vi "Asia Pump C Test.vi"() -> ()   [LabVIEW 2018, in "ASIA Pump.lvlib"]
uses:
  ASIA Pump.lvlib
  ASIA Pump/Pump Settings.ctl
panel:
  out "ASIA Pump Global 2":T1(array[cluster])
  out "Pump On?":enum16{"Off", "On", "Not Initialized"}(ring)
  out "pressure":dbl
  out "Connection Error 2":bool
  out "Connection Error":bool
  out "Pump Status Time":dbl
  out "Set Speed Time":dbl
  in  "Pump %":sgl
  in  "stop":bool
  out "PumpStatusCode":T2(ring)=enum."Idle"
  out "pumpRate":dbl format="%.2f"
  out "syringeSize":sgl
  in  "Run":bool
  in  "ASIA Pump C Settings in":T3
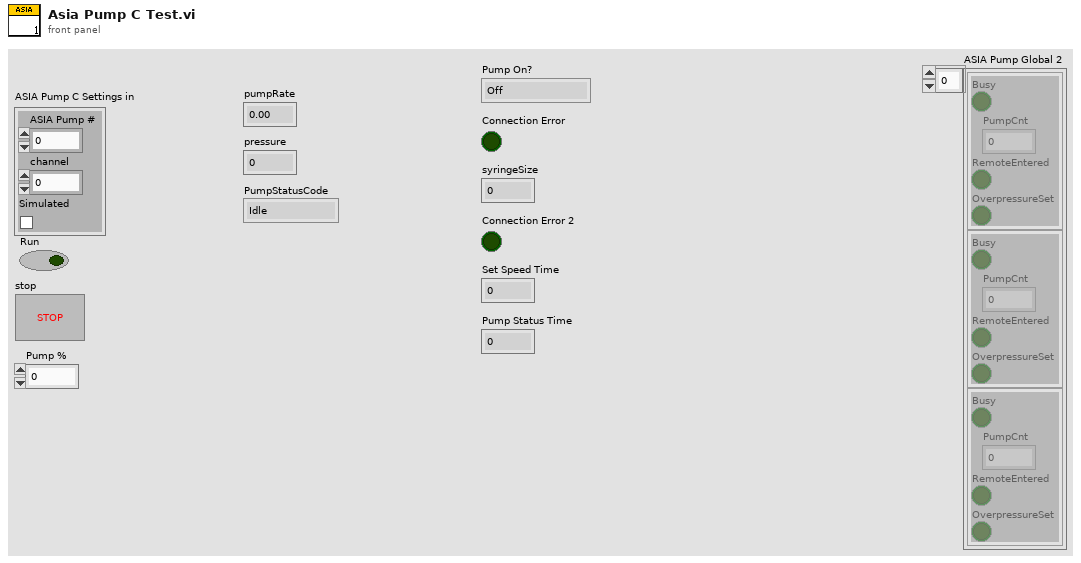
[diagram p1: front panel]
types:
  T1 = cluster{"Busy":bool, "PumpCnt":dbl, "RemoteEntered":bool, "OverpressureSet":bool}[]
  T2 = enum16{"Error", "Uninitialised", "Initialising", "Idle", "Filling", "Full", "Emptying", "Empty", "Pumping", "Default"}
  T3 = typedef "ASIA Pump.lvlib/Pump Settings.ctl" = cluster{"ASIA Pump #":i32, "channel":i32, "Simulated":bool}
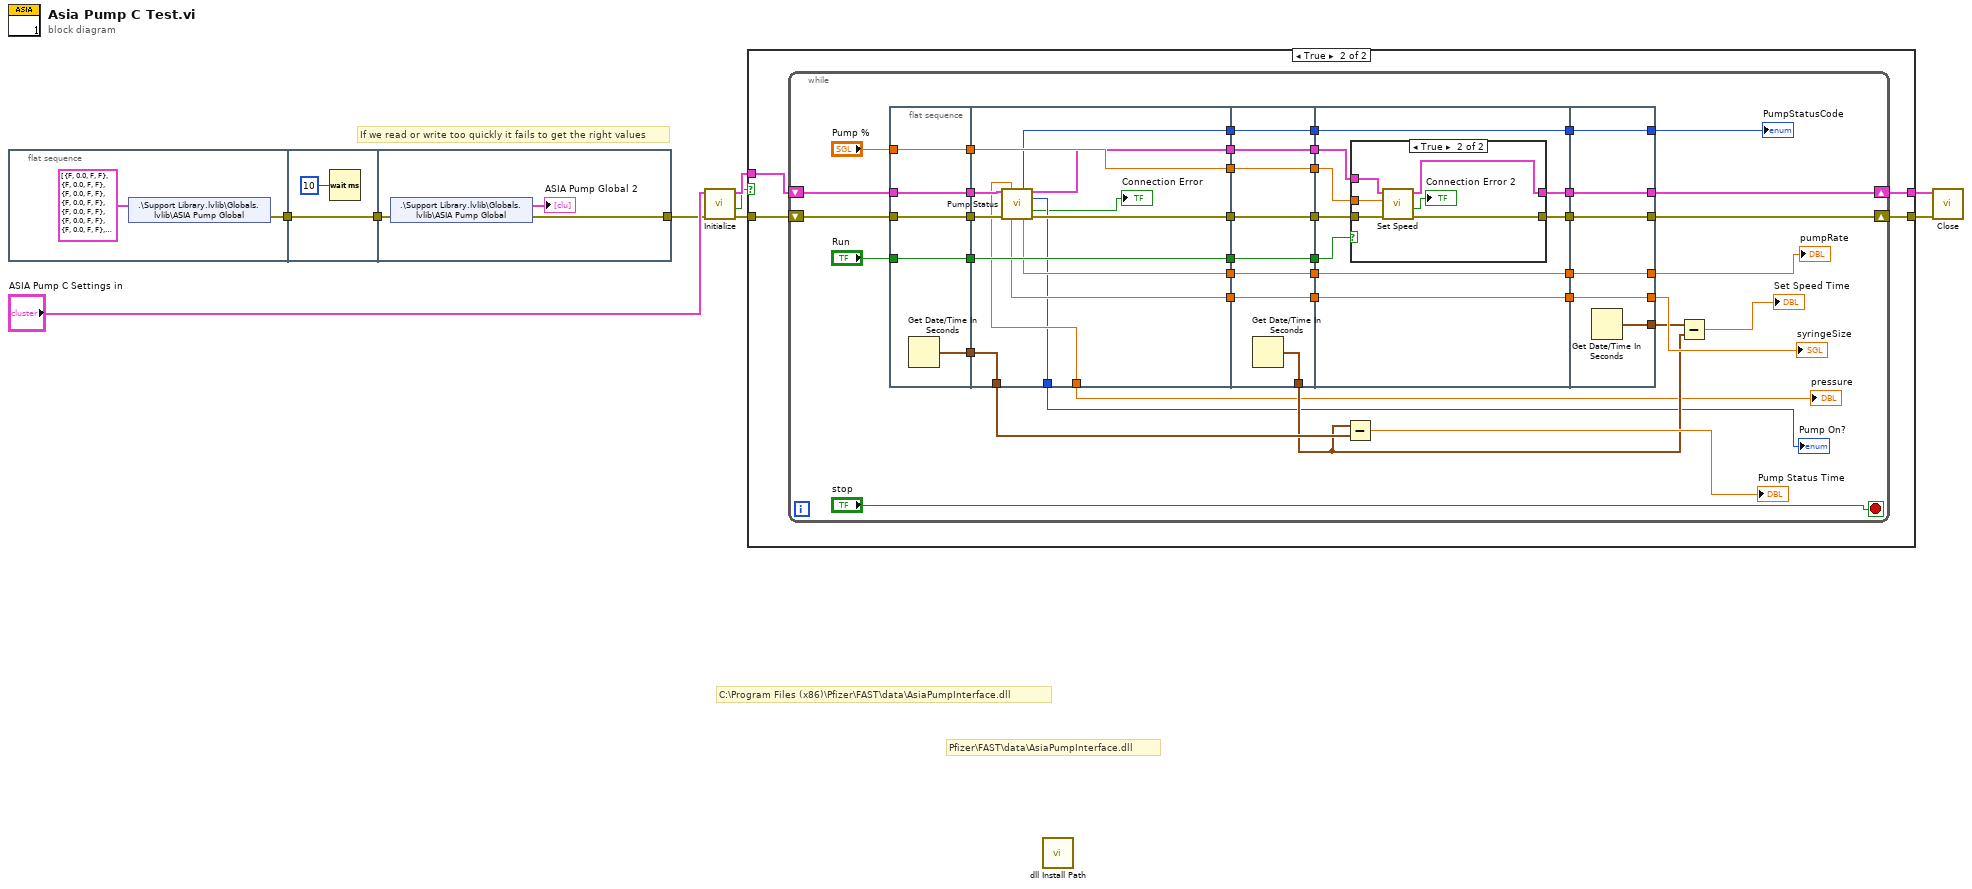
[diagram p0: block diagram]
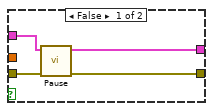
[diagram p3: hidden frame]
diagram:
  # "If we read or write too quickly it fails to get the right values"
  # "Pfizer\\FAST\\data\\AsiaPumpInterface.dll"
  # "C:\\Program Files (x86)\\Pfizer\\FAST\\data\\AsiaPumpInterface.dll"
  n1 = flat-sequence {
    tunnel: [w10] -> w9
    tunnel: w9 -> [w13]
    tunnel: [w13] -> w8
    tunnel: w8 -> [w15]
    tunnel: [w14] -> w2
    frame #0 {
      n2 = shared-variable ".\\Support Library.lvlib\\Globals.lvlib\\ASIA Pump Global"(T1 [{"Busy"=FALSE, "PumpCnt"=0.0, "RemoteEntered"=FALSE, "OverpressureSet"=FALSE}, {"Busy"=FALSE, "PumpCnt"=0.0, "RemoteEntered"=FALSE, "OverpressureSet"=FALSE}, {"Busy"=FALSE, "PumpCnt"=0.0, "RemoteEntered"=FALSE, "OverpressureSet"=FALSE}, {"Busy"=FALSE, "PumpCnt"=0.0, "RemoteEntered"=FALSE, "OverpressureSet"=FALSE}, {"Busy"=FALSE, "PumpCnt"=0.0, "RemoteEntered"=FALSE, "OverpressureSet"=FALSE}, {"Busy"=FALSE, "PumpCnt"=0.0, "RemoteEntered"=FALSE, "OverpressureSet"=FALSE}, {"Busy"=FALSE, "PumpCnt"=0.0, "RemoteEntered"=FALSE, "OverpressureSet"=FALSE}, {"Busy"=FALSE, "PumpCnt"=0.0, "RemoteEntered"=FALSE, "OverpressureSet"=FALSE}, {"Busy"=FALSE, "PumpCnt"=0.0, "RemoteEntered"=FALSE, "OverpressureSet"=FALSE}, {"Busy"=FALSE, "PumpCnt"=0.0, "RemoteEntered"=FALSE, "OverpressureSet"=FALSE}, {"Busy"=FALSE, "PumpCnt"=0.0, "RemoteEntered"=FALSE, "OverpressureSet"=FALSE}] ("ASIA Pump Global")) -> (error out=w10:errorcluster)  [unwired: 1 in]
    }
    frame #1 {
      n3 = Wait (ms)(milliseconds to wait=u32 10) -> ()  [unwired: 1 out]
    }
    frame #2 {
      n4 = shared-variable ".\\Support Library.lvlib\\Globals.lvlib\\ASIA Pump Global"(error in=w15) -> (→"ASIA Pump Global 2":T1, error out=w14:errorcluster)
    }
  }
  n5 = call "Initialize.vi"("error in (no error)"=w2, "ASIA Pump C Settings in"="ASIA Pump C Settings in") -> ("error out"=w3:errorcluster, "Initialized"=w1:bool, "ASIA Pump C Settings out"=w6:T3)  [unwired: 6 in, 1 out]
  n6 = case shown="True" w1 {
    tunnel: w6 -> [w18 w22]
    tunnel: [w18 w21] -> w5
    tunnel: [w17 w20] -> w4
    tunnel: w3 -> [w17 w19]
    frame False {
    }
    frame True {
      n7 = while {
        shift-right: [w62] -> w21
        shift-left: w22 -> [w63]
        shift-right: [w60] -> w20
        shift-left: w19 -> [w61]
        stop <- "stop" stop-if-true
        n8 = flat-sequence {
          tunnel: "Pump %" -> [w65]
          tunnel: "Run" -> [w66]
          tunnel: w61 -> [w67]
          tunnel: w63 -> [w68]
          tunnel: [w68] -> w52
          tunnel: [w67] -> w51
          tunnel: [w66] -> w50
          tunnel: [w65] -> w49
          tunnel: [w64] -> w48
          tunnel: [w74] -> w41
          tunnel: [w75] -> w39
          tunnel: [w71] -> w37
          tunnel: [w72] -> w35
          tunnel: w52 -> [w78]
          tunnel: w51 -> [w77]
          tunnel: w50 -> [w81]
          tunnel: w49 -> [w80]
          tunnel: w48 -> [w79]
          tunnel: [w81] -> w32
          tunnel: [w80] -> w30
          tunnel: [w79] -> w28
          tunnel: [w76] -> w25
          tunnel: [w70] -> w24
          tunnel: [w73] -> w23
          tunnel: w41 -> [w89]
          tunnel: [w89] -> w40
          tunnel: w39 -> [w88]
          tunnel: [w88] -> w38
          tunnel: w37 -> [w87]
          tunnel: [w87] -> w36
          tunnel: w35 -> [w86]
          tunnel: [w86] -> w34
          tunnel: [w85] -> w33
          tunnel: w32 -> [w84]
          tunnel: [w84] -> w31
          tunnel: w30 -> [w83]
          tunnel: [w83] -> w29
          tunnel: [w82] -> w26
          tunnel: w23 -> [w85]
          tunnel: w40 -> [w94]
          tunnel: [w91] -> w46
          tunnel: w38 -> [w93]
          tunnel: [w90] -> w45
          tunnel: w36 -> [w98]
          tunnel: [w98] -> w44
          tunnel: w34 -> [w97]
          tunnel: [w97] -> w43
          tunnel: w33 -> [w96]
          tunnel: [w96] -> w42
          tunnel: w31 -> [w95]
          tunnel: w29 -> [w92]
          tunnel: [w110] -> w56
          tunnel: [w111] -> w57
          tunnel: [w112] -> w58
          tunnel: [w113] -> w60
          tunnel: [w114] -> w62
          tunnel: w46 -> [w114]
          tunnel: w45 -> [w113]
          tunnel: w44 -> [w112]
          tunnel: w43 -> [w111]
          tunnel: w42 -> [w110]
          tunnel: [w109] -> w47
          frame #0 {
            n9 = Get Date/Time In Seconds() -> (seconds since 1Jan1904=w64:timestamp)
          }
          frame #1 {
            n10 = call "Pump Status.vi"("ASIA Pump C Settings in"=w78, "error in (no error)"=w77) -> ("pressure"=w76:dbl, "PumpStatusCode"=w73:T2, "ASIA Pump C Settings out"=w74:T3, "Pump On?"=w70:enum16{"Off", "On", "Not Initialized"}, "Connection Error"=→"Connection Error":bool, "syringeSize (ml)"=w71:sgl, "pumpRate"=w72:dbl, "error out"=w75:errorcluster)  [unwired: 5 in, 1 out]
          }
          frame #2 {
            n11 = Get Date/Time In Seconds() -> (seconds since 1Jan1904=w82:timestamp)
          }
          frame #3 {
            n12 = case shown="True" w95 {
              tunnel: w94 -> [w100 w105]
              tunnel: [w102 w108] -> w91
              tunnel: w93 -> [w99 w104]
              tunnel: [w101 w107] -> w90
              tunnel: w92 -> [_ w106]
              frame False {
                n13 = call "Pause.vi"("error in (no error)"=w99, "ASIA Pump C Settings in"=w100) -> ("error out"=w101:errorcluster, "ASIA Pump C Settings out"=w102:T3)  [unwired: 7 in, 1 out]
              }
              frame True {
                n14 = call "Set Speed.vi"("error in (no error)"=w104, "Pump %"=w106, "ASIA Pump C Settings in"=w105) -> ("error out"=w107:errorcluster, "Connection Error"=→"Connection Error 2":bool, "ASIA Pump C Settings out"=w108:T3)  [unwired: 6 in]
              }
            }
          }
          frame #4 {
            n15 = Get Date/Time In Seconds() -> (seconds since 1Jan1904=w109:timestamp)
          }
        }
        n16 = Subtract(x=w26, y=w28) -> (x-y=→"Pump Status Time":dbl)
        n17 = Subtract(x=w47, y=w26) -> (x-y=→"Set Speed Time":dbl)
        "syringeSize" <- w58
        "pumpRate" <- w57
        "PumpStatusCode" <- w56
        "pressure" <- w25
        "Pump On?" <- w24
      }
    }
  }
  n18 = call "dll Install Path.vi"() -> ()  [unwired: 11 in, 1 out]
  n19 = call "Close.vi"("error in (no error)"=w4, "ASIA Pump C"=w5) -> ()  [unwired: 7 in, 3 out]
